vi "enqueue_proc_img.vi"(2 "Proc Img Data In":T2, 7 "Proc Img Notifier In":T1) -> (8 "Proc Img Notifier Out":T1)   [LabVIEW 2023]
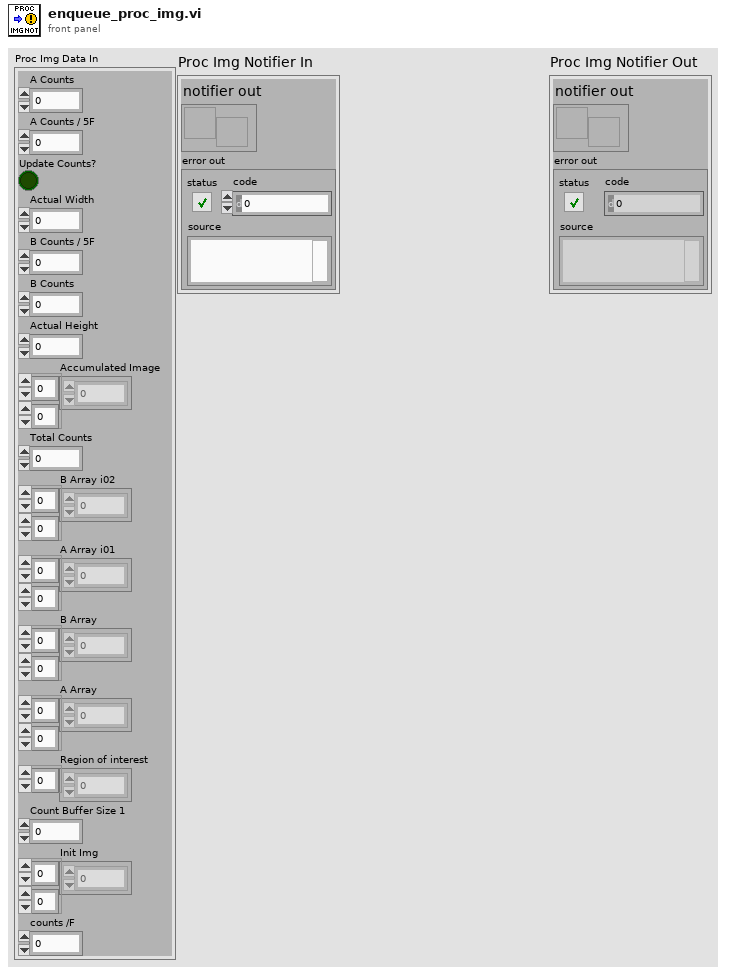
[diagram p1: front panel]
types:
  T1 = cluster{"notifier out":refnum<notifier>, "error out":errorcluster}
  T2 = cluster{"A Counts":i32, "A Counts / 5F":dbl, "Update Counts?":bool, "Actual Width":u32, "B Counts / 5F ":dbl, "B Counts":i32, "Actual Height":u32, "Accumulated Image ":i16[][], "Total Counts":i32, "B Array i02":sgl[][], "A Array i01":sgl[][], "B Array":i16[][], "A Array":i16[][], "Region of interest":i32[], "Count Buffer Size 1":i32, "Init Img":i16[][], "counts /F":i16}
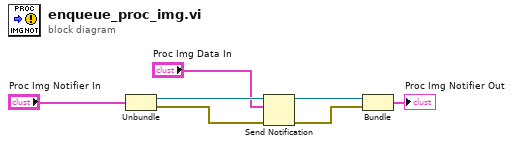
[diagram p0: block diagram]
diagram:
  n1 = Unbundle("Proc Img Notifier In") -> ("notifier out"=w6:refnum<notifier>, "error out"=w5:errorcluster)
  n2 = Send Notification(notification="Proc Img Data In", notifier=w6, error in (no error)=w5) -> (notifier out=w4:refnum<notifier>, error out=w3:errorcluster)
  n3 = Bundle("notifier out"=w4, "error out"=w3) -> (→"Proc Img Notifier Out":T1)  [unwired: 1 in]
